vi "getCategoryDefaultAmount.vi"(8 "error in (no error)":errorcluster, 10 "Name":string, 11 "Account History in":refnum<class "Account History.lvclass">) -> (0 "error out":errorcluster, 2 "Default Amount":dbl, 3 "Account History out":refnum<class "Account History.lvclass">)   [LabVIEW 2018, in "Account History.lvclass"]
uses:
  Account History.lvclass
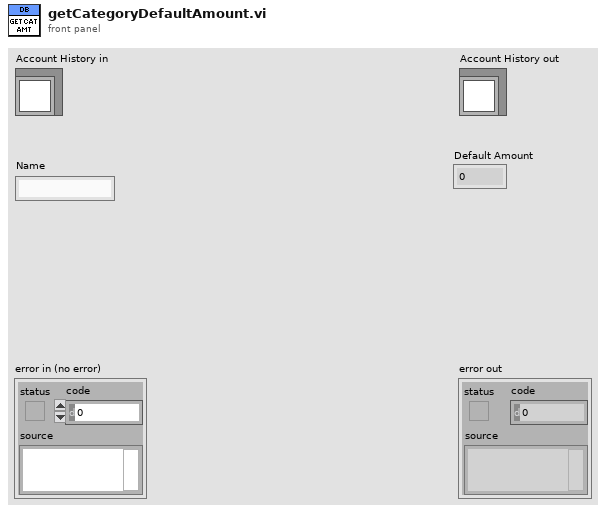
[diagram p1: front panel]
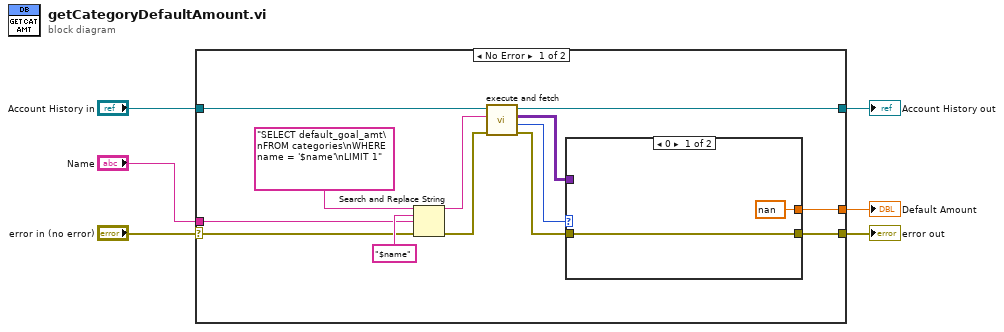
[diagram p0: block diagram]
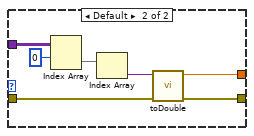
[diagram p2: hidden frame]
diagram:
  n1 = case shown="No Error" "error in (no error)" {
    selector: "error in (no error)" -> [w10 w30]
    tunnel: [w7 w30] -> w5
    tunnel: [w11 w29] -> w3
    tunnel: "Account History in" -> [w12 w29]
    tunnel: "Name" -> [w9 _]
    tunnel: [w8 _] -> w1
    frame No Error {
      n2 = Search and Replace String(input string="SELECT default_goal_amt\nFROM categories\nWHERE name = '$name'\nLIMIT 1", search string="$name", replace string=w9, error in=w10) -> (result string=w17:string, error out=w16:errorcluster)  [unwired: 4 in, 2 out]
      n3 = call "execute and fetch.vi"("error in (no error)"=w16, "SQL query"=w17, "Database in"=w12) -> ("error out"=w14:errorcluster, "Num records"=w13:i32, "recordset data"=w15:variant[][], "Database out"=w11:refnum<class "Account History.lvclass">)  [unwired: 5 in]
      n4 = case shown="0" w13 {
        tunnel: w15 -> [_ w28]
        tunnel: w14 -> [w21 w24]
        tunnel: [nan ("type") w23] -> w8
        tunnel: [w21 w22] -> w7
        frame 0 {
        }
        frame Default {
          n5 = Index Array(array=w28, index (row)=0) -> (element=w26:variant[])  [unwired: 1 in]
          n6 = Index Array(array=w26) -> (element=w25:variant)  [unwired: 1 in]
          n7 = call "toDouble.vi"("error in (no error)"=w24, "Value"=w25) -> ("error out"=w22:errorcluster, "type"=w23:dbl)  [unwired: 8 in]
        }
      }
    }
    frame Error {
    }
  }
  "error out" <- w5
  "Account History out" <- w3
  "Default Amount" <- w1
